vi "Attempt to resolve locally.vi"(8 "error in (no error)":errorcluster, 11 "address":refnum<class "Hostname Network Address.lvclass">) -> (0 "error out":errorcluster, 3 "addresses out":refnum<class "Generic Network Address.lvclass">[](array[class]))   [LabVIEW 2020, in "NI_WFCN.lvlib" / "Hostname Network Address.lvclass"]
doc: "Use local facilities to resolve this address into the address which should be resolved next. For IP addresses, this typically does nothing. If a hostname is in /etc/hosts, this will look up its IP and return it. For DNS hostnames, this will return a DNS nameserver IP."
uses:
  <vilib>/net/WFCN/Addressing/Hostname Network Address/Hostname Network Address.lvclass
  e:/builds/penguin/labview/branches/2020/dev/dist/vi.lib/net/WFCN/Addressing/Generic Network Address/Generic Network Address.lvclass
  <vilib>/net/WFCN/Addressing/Generic Network Address/Generic Network Address.lvclass
  <vilib>/net/WFCN/Addressing/Hostname Network Address/Hostname Network Address.lvclass/Hostname Network Address.ctl
  <vilib>/net/WFCN/Addressing/IPv4 Network Address/IPv4 Network Address.lvclass/IPv4 Network Address.ctl
  <vilib>/net/WFCN/Addressing/Generic Network Address/Generic Network Address.lvclass/Generic Network Address.ctl
  <vilib>/net/WFCN/Addressing/Hostname Network Address/Search etc-hosts contents.vi
  <vilib>/net/WFCN/Addressing/Hostname Network Address/Windows Scan DNS Config.vi
  <vilib>/net/WFCN/Addressing/Generic Network Address/Parse.vi
  <vilib>/Utility/error.llb/Clear Errors.vi
  <vilib>/net/WFCN/Addressing/Hostname Network Address/Create from string.vi
  <vilib>/net/WFCN/Utility/Is IPv4 address.vi
  <vilib>/net/WFCN/Addressing/Generic Network Address/Create for unparsable.vi
  <vilib>/net/WFCN/Utility/Is hostname mDNS.vi
  <vilib>/dlg_ctls.llb/Space Constant.vi
  <vilib>/net/WFCN/Addressing/IPv4 Network Address/IPv4 Network Address.lvclass
  <vilib>/net/WFCN/Addressing/mDNS Hostname Network Address/mDNS Hostname Network Address.lvclass
  e:/builds/penguin/labview/branches/2020/dev/dist/vi.lib/net/WFCN/Addressing/Hostname Network Address/Hostname Network Address.lvclass
  <vilib>/Utility/error.llb/Error Cluster From Error Code.vi
  <vilib>/net/WFCN/Addressing/Hostname Network Address/Windows run ipconfig.vi
  <vilib>/net/WFCN/Addressing/Hostname Network Address/Parse ipconfig.vi
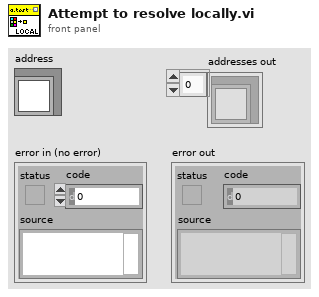
[diagram p1: front panel]
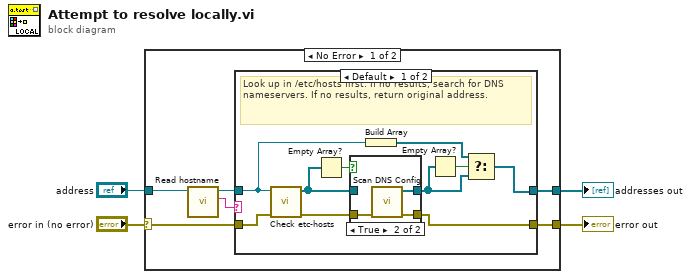
[diagram p0: block diagram]
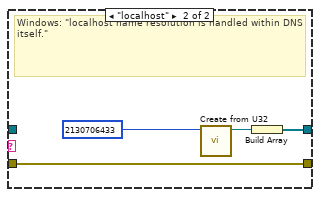
[diagram p3: hidden frame]
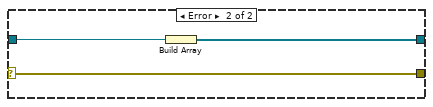
[diagram p4: hidden frame]
diagram:
  n1 = case shown="No Error" "error in (no error)" {
    selector: "error in (no error)" -> [w6 w32]
    tunnel: [w10 w30] -> w1
    tunnel: [w9 w32] -> w4
    tunnel: "address" -> [w8 w31]
    frame No Error {
      n2 = call <vilib>:"Read hostname.vi"("address"=w8) -> ("hostname"=w5:string, "address out"=w7:refnum<class "Hostname Network Address.lvclass">)  [unwired: 9 in]
      n3 = case shown="Default" w5 {
        tunnel: w6 -> [w20 w28]
        tunnel: [w16 w26] -> w10
        tunnel: [w15 w28] -> w9
        tunnel: w7 -> [w18 _]
        frame Default {
          # "Look up in /etc/hosts first. If no results, search for DNS nameservers. If no results, return original address."
          n4 = call <vilib>:"Check etc-hosts.vi"("error in"=w20, "address"=w18) -> ("error out"=w19:errorcluster, "resolved addresses"=w13:refnum<class "Generic Network Address.lvclass">[])  [unwired: 8 in]
          n5 = Empty Array?(array=w13) -> (empty?=w14:bool)
          n6 = case shown="True" w14 {
            tunnel: [w22 w23] -> w11
            tunnel: w19 -> [w21 w25]
            tunnel: [w21 w24] -> w15
            tunnel: w13 -> [w22 _]
            frame False {
            }
            frame True {
              n7 = call <vilib>:"Scan DNS Config.vi"("error in (no error)"=w25) -> ("error out"=w24:errorcluster, "DNS server addresses"=w23:refnum<class "Generic Network Address.lvclass">[])  [unwired: 8 in, 1 out]
            }
          }
          n8 = Build Array(w18) -> (w17:refnum<class "Hostname Network Address.lvclass">[])
          n9 = Empty Array?(array=w11) -> (empty?=w12:bool)
          n10 = Select(t=w17, s=w12, f=w11) -> (s? t:f=w16:refnum<class "Generic Network Address.lvclass">[])
        }
        frame "localhost" {
          # "Windows: \"localhost name resolution is handled within DNS itself.\""
          n11 = call <vilib>:"Create from U32.vi"("address U32"=u32 2130706433 ("address")) -> ("address out"=w27:refnum<class "IPv4 Network Address.lvclass">)  [unwired: 10 in]
          n12 = Build Array(w27) -> (w26:refnum<class "IPv4 Network Address.lvclass">[])
        }
      }
    }
    frame Error {
      n13 = Build Array(w31) -> (w30:refnum<class "Hostname Network Address.lvclass">[])
    }
  }
  "error out" <- w4
  "addresses out" <- w1
